vi "Set Focus Position.vi"(8 "error in (no error)":errorcluster, 11 "TE2000 in":refnum<class "TE2000.lvclass">) -> (0 "error out":errorcluster, 3 "TE2000 out":refnum<class "TE2000.lvclass">)   [LabVIEW 2014, in "TE2000.lvlib" / "TE2000.lvclass"]
uses:
  TE2000.lvclass
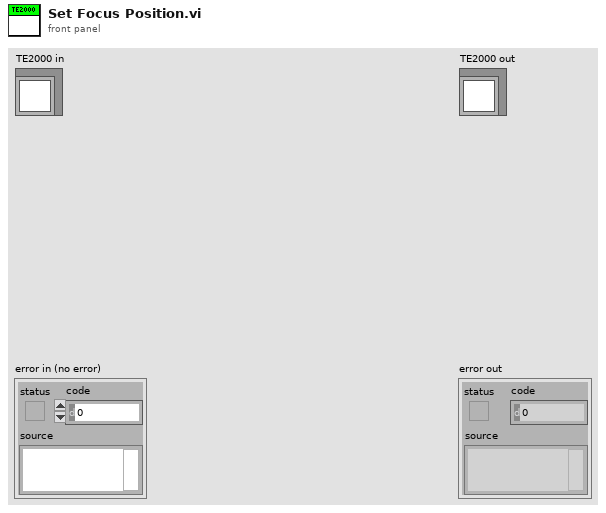
[diagram p1: front panel]
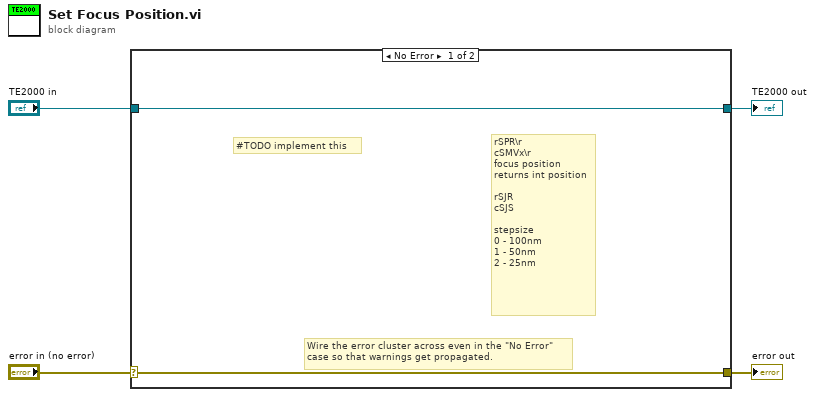
[diagram p0: block diagram]
diagram:
  n1 = case shown="No Error" "error in (no error)" {
    selector: "error in (no error)" -> [w5 w8]
    tunnel: [w5 w8] -> w3
    tunnel: [w6 w7] -> w1
    tunnel: "TE2000 in" -> [w6 w7]
    frame No Error {
      # "rSPR\\r\ncSMVx\\r\nfocus position\nreturns int position\n\nrSJR\ncSJS\n\nstepsize\n0 - 100nm\n1 - 50nm\n2 - 25nm"
      # "#TODO implement this"
      # "Wire the error cluster across even in the \"No Error\"\ncase so that warnings get propagated."
    }
    frame Error {
    }
  }
  "error out" <- w3
  "TE2000 out" <- w1
